vi "CALC GEAR RATIO SPEEDS.vi"(8 "error in (no error)":errorcluster) -> (0 "error out":errorcluster, 1 "Vel ratios":T1, 2 "K LOADER":dbl format="%#_13g", 3 "K INTAKE":dbl format="%#_13g")   [LabVIEW 2023]
uses:
  Global INIT.vi
  ctrl defs/ctrl MOTOR SELECT.ctl
panel:
  out "SHOOTER MOTORS":T2 items=["REV NEO"=5676, "REV NEO 550"=11000, "VEX Falcon"=6380, "WC Kraken"=6000]
  out "SHOOTER ratio":dbl=4.0
  out "SHOOTER\n(rpm)":dbl
  out "R shooter (in)":dbl
  out "Vel SHOOTER\n(in/s) 2":dbl format="%_4f"
  out "INTAKE MOTOR":T2 items=["REV NEO"=5676, "REV NEO 550"=11000, "VEX Falcon"=6380, "WC Kraken"=6000]
  out "LOADER MOTORS":T2 items=["REV NEO"=5676, "REV NEO 550"=11000, "VEX Falcon"=6380, "WC Kraken"=6000]
  out "Vel LOADER\n(in/s)":dbl format="%_4f"
  out "R loader (in)":dbl
  out "LOADER\n(rpm)":dbl
  out "LOADER ratio":dbl=4.0
  out "INTAKE ratio":dbl=4.0
  out "R LG (in)":dbl format="%.3f"
  out "R SM (in)":dbl format="%.3f"
  out "large wheel\n(in/s)":dbl format="%_4f"
  out "small wheel\n(in/s)":dbl format="%_4f"
  out "INTAKE LG WHEEL\n(rpm)":dbl format="%#.3f"
  out "INTAKE SM WHEEL\n(rpm)":dbl format="%#.3f"
  out "INTAKE GEAR TRAIN\nGEAR RATIO\nto SM WHEEL":dbl
  out "INTAKE GEAR TRAIN\nGEAR RATIO\nto LRG WHEEL":dbl
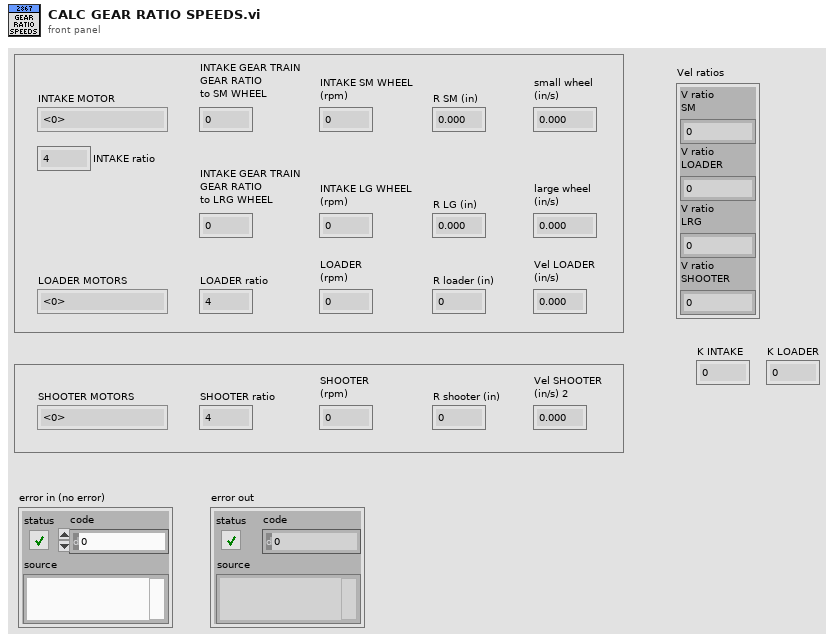
[diagram p1: front panel]
types:
  T1 = cluster{"V ratio\nSM":dbl, "V ratio\nLOADER":dbl, "V ratio\nLRG":dbl, "V ratio\nSHOOTER":dbl}
  T2 = typedef "ctrl MOTOR SELECT.ctl" = i16
  T3 = typedef "ctrl swerve motor.ctl" = cluster{"description":string, "MOTOR SELECT":T2, "Installed?":bool, "CAN ID":u8, "refnum name":string, "Invert":bool, "Idle Mode":T4, "Current limiting":T5}
  T4 = typedef "Spark MAX Idle Mode.ctl" = enum16{"Coast", "Brake"}
  T5 = typedef "ctrl Spark MAX current limiting.ctl" = cluster{"Linearized":bool, "Free Speed (A)":dbl, "Primay (A)":dbl, "Limit RPM (0)":u32}
  T6 = typedef "ctrl DEFINE GEAR.ctl" = cluster{"DP":dbl, "TEETH":i16, "DIAM (in)":dbl, "rev":bool, "ratio":dbl}
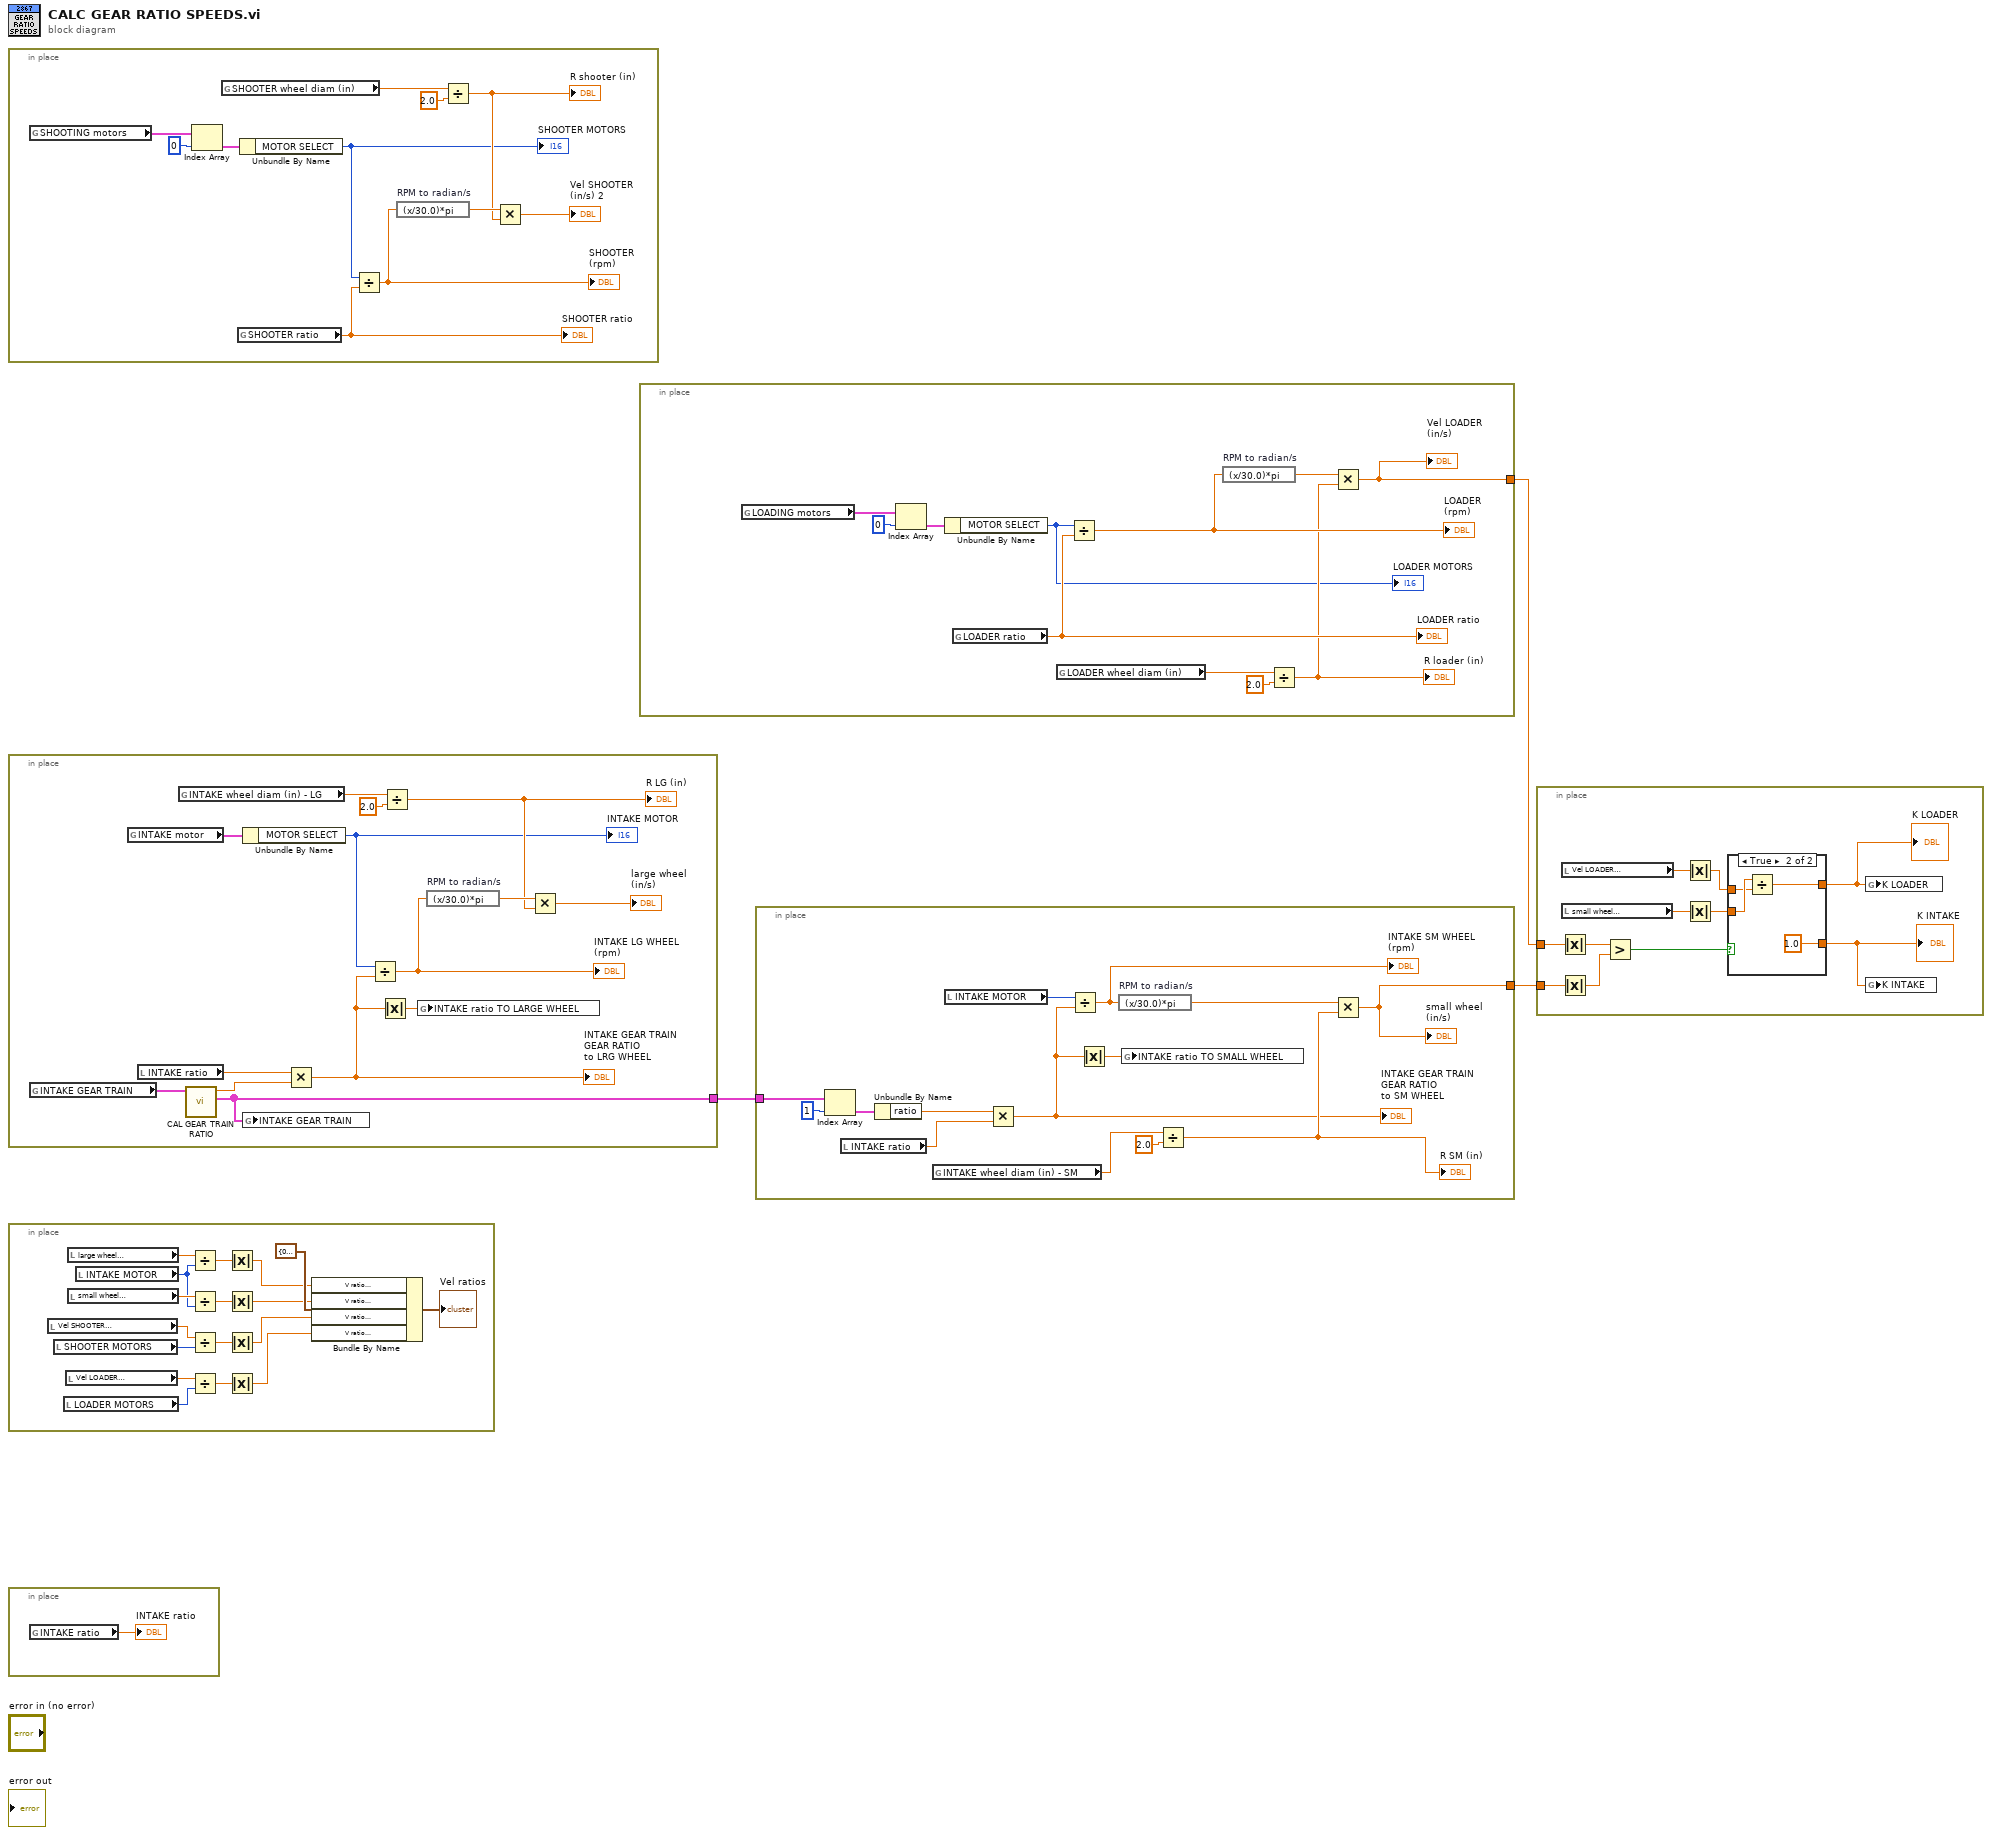
[diagram p0: block diagram]
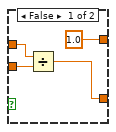
[diagram p2: hidden frame]
diagram:
  n1 = in-place {
    n2 = global read "Global INIT.vi" "SHOOTING motors"() -> (w7:T3[])
    n3 = Index Array(array=w7, index=0) -> (element=w5:T3)
    n4 = global read "Global INIT.vi" "SHOOTER wheel diam (in)"() -> (w14:dbl)
    n5 = global read "Global INIT.vi" "SHOOTER ratio"() -> (w8:dbl)
    "SHOOTER ratio" <- w8
    n6 = Unbundle By Name(w5) -> ("MOTOR SELECT"=w4:T2)
    "SHOOTER MOTORS" <- w4
    n7 = Divide(x=w4, y=w8) -> (x/y=w12:dbl)
    "SHOOTER\n(rpm)" <- w12
    n8 = expression code="(x/30.0)*pi" "RPM to radian/s"(w12) -> (w11:dbl)
    n9 = Divide(x=w14, y=2.0) -> (x/y=w10:dbl)
    "R shooter (in)" <- w10
    n10 = Multiply(x=w11, y=w10) -> (x*y=→"Vel SHOOTER\n(in/s) 2":dbl)
  }
  n11 = in-place {
    in-place-border: [w20] -> w3
    n12 = global read "Global INIT.vi" "INTAKE GEAR TRAIN"() -> (w28:T6[])
    n13 = global read "Global INIT.vi" "INTAKE motor"() -> (w17:T3)
    n14 = local read "INTAKE ratio"() -> (w18:dbl)
    n15 = global read "Global INIT.vi" "INTAKE wheel diam (in) - LG"() -> (w23:dbl)
    n16 = call "CAL GEAR TRAIN RATIO.vi"("GEAR TRAIN definition"=w28) -> ("GEAR TRAIN updated"=w20:T6[], "GEAR RATIO"=w27:dbl)  [unwired: 9 in]
    n17 = Unbundle By Name(w17) -> ("MOTOR SELECT"=w16:T2)
    "INTAKE MOTOR" <- w16
    n18 = global write "Global INIT.vi" "INTAKE GEAR TRAIN"(w20) -> ()
    n19 = Multiply(x=w18, y=w27) -> (x*y=w19:dbl)
    "INTAKE GEAR TRAIN\nGEAR RATIO\nto LRG WHEEL" <- w19
    n20 = Divide(x=w16, y=w19) -> (x/y=w21:dbl)
    "INTAKE LG WHEEL\n(rpm)" <- w21
    n21 = Absolute Value(x=w19) -> (abs(x)=w15:dbl)
    n22 = Divide(x=w23, y=2.0) -> (x/y=w25:dbl)
    "R LG (in)" <- w25
    n23 = global write "Global INIT.vi" "INTAKE ratio TO LARGE WHEEL"(w15) -> ()
    n24 = expression code="(x/30.0)*pi" "RPM to radian/s"(w21) -> (w26:dbl)
    n25 = Multiply(x=w26, y=w25) -> (x*y=→"large wheel\n(in/s)":dbl)
  }
  n26 = in-place {
    n27 = local read "Vel SHOOTER\n(in/s) 2"() -> (w36:dbl)
    n28 = local read "SHOOTER MOTORS"() -> (w35:T2)
    n29 = local read "LOADER MOTORS"() -> (w43:T2)
    n30 = local read "Vel LOADER\n(in/s)"() -> (w44:dbl)
    n31 = local read "large wheel\n(in/s)"() -> (w38:dbl)
    n32 = local read "small wheel\n(in/s)"() -> (w45:dbl)
    n33 = local read "INTAKE MOTOR"() -> (w39:T2)
    n34 = Divide(x=w38, y=w39) -> (x/y=w40:dbl)
    n35 = Divide(x=w45, y=w39) -> (x/y=w42:dbl)
    n36 = Divide(x=w36, y=w35) -> (x/y=w37:dbl)
    n37 = Divide(x=w44, y=w43) -> (x/y=w41:dbl)
    n38 = Absolute Value(x=w40) -> (abs(x)=w32:dbl)
    n39 = Absolute Value(x=w42) -> (abs(x)=w31:dbl)
    n40 = Absolute Value(x=w37) -> (abs(x)=w30:dbl)
    n41 = Absolute Value(x=w41) -> (abs(x)=w29:dbl)
    n42 = Bundle By Name(cluster=T1 {"V ratio\nSM"=0.026179938779914945, "V ratio\nLOADER"=0.03599741582238305, "V ratio\nLRG"=0.05235987755982989, "V ratio\nSHOOTER"=0.05235987755982989} ("Cluster"), "V ratio\nLRG"=w32, "V ratio\nSM"=w31, "V ratio\nSHOOTER"=w30, "V ratio\nLOADER"=w29) -> (→"Vel ratios":T1)
  }
  n43 = in-place {
    n44 = global read "Global INIT.vi" "INTAKE ratio"() -> (→"INTAKE ratio":dbl)
  }
  n45 = in-place {
    in-place-border: [w47] -> w2
    n46 = global read "Global INIT.vi" "LOADING motors"() -> (w50:T3[])
    n47 = Index Array(array=w50, index=0) -> (element=w51:T3)
    n48 = Unbundle By Name(w51) -> ("MOTOR SELECT"=w48:T2)
    "LOADER MOTORS" <- w48
    n49 = global read "Global INIT.vi" "LOADER ratio"() -> (w57:dbl)
    "LOADER ratio" <- w57
    n50 = global read "Global INIT.vi" "LOADER wheel diam (in)"() -> (w56:dbl)
    n51 = Divide(x=w48, y=w57) -> (x/y=w54:dbl)
    "LOADER\n(rpm)" <- w54
    n52 = expression code="(x/30.0)*pi" "RPM to radian/s"(w54) -> (w53:dbl)
    n53 = Divide(x=w56, y=2.0) -> (x/y=w52:dbl)
    "R loader (in)" <- w52
    n54 = Multiply(x=w53, y=w52) -> (x*y=w47:dbl)
    "Vel LOADER\n(in/s)" <- w47
  }
  n55 = in-place {
    in-place-border: w3 -> [w66]
    in-place-border: [w60] -> w1
    n56 = Index Array(array=w66, index=1) -> (element=w64:T6)
    n57 = local read "INTAKE ratio"() -> (w62:dbl)
    n58 = Unbundle By Name(w64) -> ("ratio"=w61:dbl)
    n59 = global read "Global INIT.vi" "INTAKE wheel diam (in) - SM"() -> (w70:dbl)
    n60 = local read "INTAKE MOTOR"() -> (w59:T2)
    n61 = Multiply(x=w61, y=w62) -> (x*y=w63:dbl)
    "INTAKE GEAR TRAIN\nGEAR RATIO\nto SM WHEEL" <- w63
    n62 = Divide(x=w59, y=w63) -> (x/y=w71:dbl)
    "INTAKE SM WHEEL\n(rpm)" <- w71
    n63 = Absolute Value(x=w63) -> (abs(x)=w58:dbl)
    n64 = expression code="(x/30.0)*pi" "RPM to radian/s"(w71) -> (w68:dbl)
    n65 = global write "Global INIT.vi" "INTAKE ratio TO SMALL WHEEL"(w58) -> ()
    n66 = Divide(x=w70, y=2.0) -> (x/y=w67:dbl)
    "R SM (in)" <- w67
    n67 = Multiply(x=w68, y=w67) -> (x*y=w60:dbl)
    "small wheel\n(in/s)" <- w60
  }
  n68 = in-place {
    in-place-border: w2 -> [w81]
    in-place-border: w1 -> [w80]
    n69 = Absolute Value(x=w81) -> (abs(x)=w77:dbl)
    n70 = Absolute Value(x=w80) -> (abs(x)=w76:dbl)
    n71 = local read "Vel LOADER\n(in/s)"() -> (w79:dbl)
    n72 = local read "small wheel\n(in/s)"() -> (w78:dbl)
    n73 = Greater?(x=w77, y=w76) -> (0:w82:bool)
    n74 = Absolute Value(x=w79) -> (abs(x)=w75:dbl)
    n75 = Absolute Value(x=w78) -> (abs(x)=w74:dbl)
    n76 = case shown="True" w82 {
      tunnel: w75 -> [w84 w87]
      tunnel: [1.0 w90] -> w73
      tunnel: [w85 1.0] -> w72
      tunnel: w74 -> [w83 w88]
      frame False {
        n77 = Divide(x=w84, y=w83) -> (x/y=w85:dbl)
      }
      frame True {
        n78 = Divide(x=w88, y=w87) -> (x/y=w90:dbl)
      }
    }
    "K INTAKE" <- w72
    "K LOADER" <- w73
    n79 = global write "Global INIT.vi" "K LOADER"(w73) -> ()
    n80 = global write "Global INIT.vi" "K INTAKE"(w72) -> ()
  }
